vi "Ejercicio_12_nodo_de_propiedad_fill_color.vi"() -> ()   [LabVIEW 2020]
panel:
  out "Waveform Chart":dbl(graph)
  in  "Cadena caracteres":string
  in  "Posicion Horizontal":dbl(slide) scale=0.0..10.0
  in  "Posicion vertical":dbl(slide) scale=0.0..10.0
  in  "Boolean":bool
  in  "Deshabilitar":bool
  in  "Limite":dbl
  in  "stop":bool
  out "Tank":dbl(slide) scale=0.0..10.0
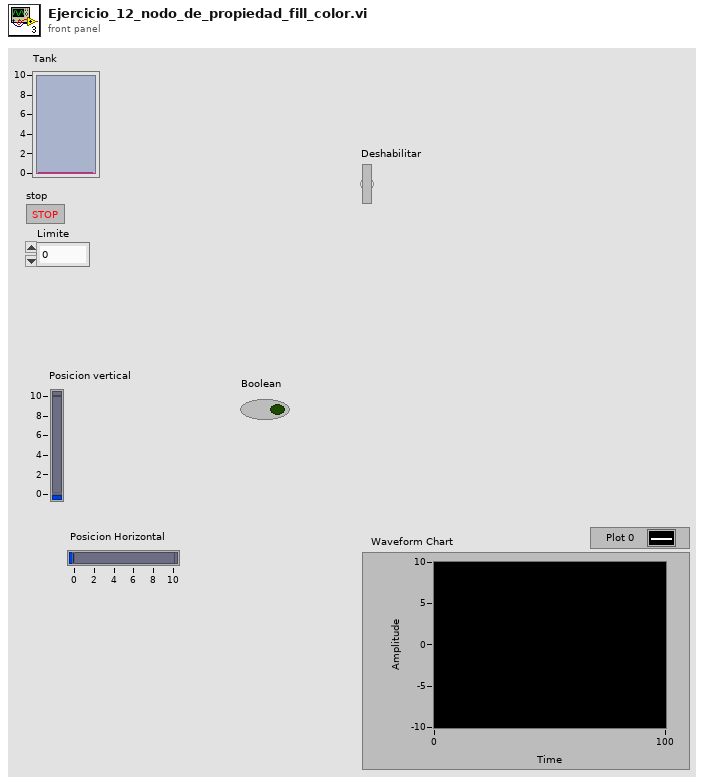
[diagram p1: front panel]
types:
  T1 = cluster{"Posicion vertical":dbl, "Posicion Horizontal ":dbl}
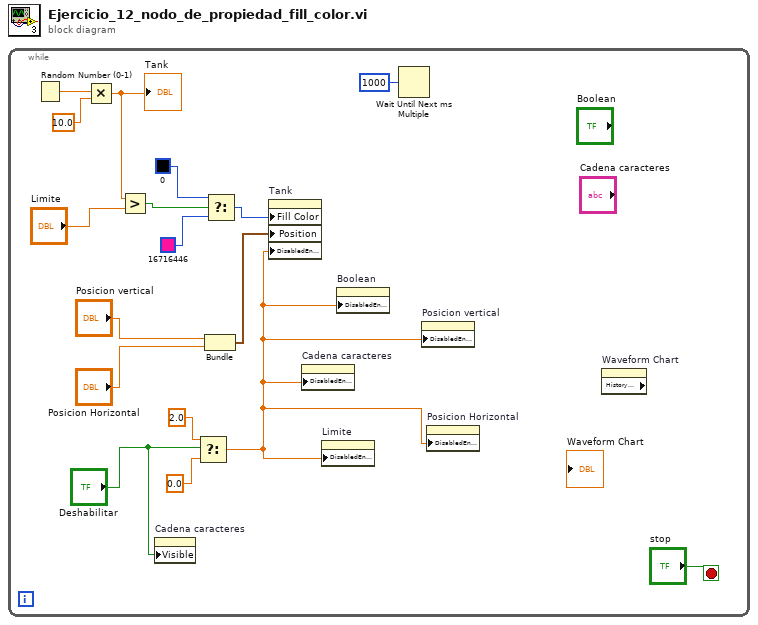
[diagram p0: block diagram]
diagram:
  n1 = while {
    stop <- "stop" stop-if-true
    n2 = Random Number (0-1)() -> (number: 0 to 1=w16:dbl)
    n3 = Multiply(x=w16, y=10.0) -> (x*y=w13:dbl)
    "Tank" <- w13
    n4 = Greater?(x=w13, y="Limite") -> (0:w11:bool)
    n5 = property on="Cadena caracteres" class="Str"("Visible"="Deshabilitar") -> ()  [unwired: 2 in, 2 out]
    n6 = Select(t=2.0, s="Deshabilitar", f=0.0) -> (s? t:f=w2:dbl)
    n7 = Bundle("Posicion vertical"="Posicion vertical", "Posicion Horizontal"="Posicion Horizontal") -> (w3:T1)  [unwired: 1 in]
    n8 = Select(t=u32 0, s=w11, f=u32 16716446) -> (s? t:f=w8:u32)
    n9 = property on="Tank" class="Slide (strict)"("Fill Color"=w8, "Position"=w3, "DisabledEnum"=w2) -> ()  [unwired: 2 in, 2 out]
    n10 = property on="Cadena caracteres" class="Str"("DisabledEnum"=w2) -> ()  [unwired: 2 in, 2 out]
    n11 = property on="Limite" class="DigNum (strict)"("DisabledEnum"=w2) -> ()  [unwired: 2 in, 2 out]
    n12 = property on="Boolean" class="Bool (strict)"("DisabledEnum"=w2) -> ()  [unwired: 2 in, 2 out]
    n13 = Wait Until Next ms Multiple(millisecond multiple=u32 1000) -> ()  [unwired: 1 out]
    n14 = property on="Posicion vertical" class="Slide (strict)"("DisabledEnum"=w2) -> ()  [unwired: 2 in, 2 out]
    n15 = property on="Posicion Horizontal" class="Slide (strict)"("DisabledEnum"=w2) -> ()  [unwired: 2 in, 2 out]
    n16 = property on="Waveform Chart" class="WFChart (strict)" props=["History Data"]() -> ()  [unwired: 2 in, 3 out]
  }
